vi "U-751 XY Stage Engine.vi"(0 "Notifier Name":string, 11 "COM Port":string[](array[string])) -> ()   [LabVIEW 2016]
uses:
  Stages Controls/Stage Notifier Element.ctl
  Stages Controls/Stage Actions.ctl
  Stages Controls/Stage Status.ctl
panel:
  in  "Quit":bool
  in  "Halt":bool
  in  "Home":bool
  in  "Get Position":bool
  in  "Y Position (µm)":dbl format="%#_4g"
  in  "X Position (µm)":dbl format="%#_4g"
  in  "XY Step Size (µm)":dbl format="%#_4g"
  in  "Up":bool
  in  "Down":bool
  in  "Left":bool
  in  "Right":bool
  in  "ReInitialize":bool
  in  "Error":bool
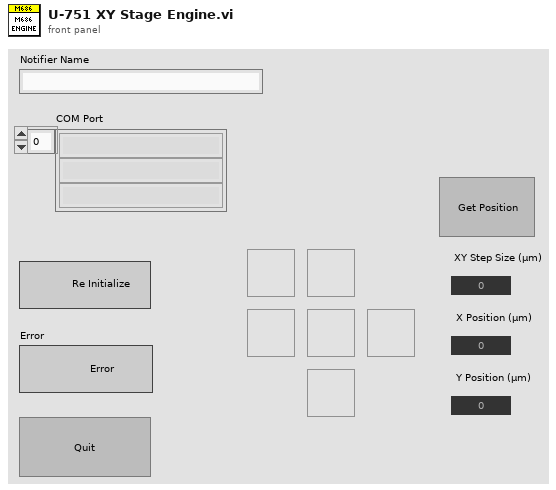
[diagram p1: front panel]
types:
  T1 = typedef "Stage Notifier Element.ctl" = cluster{"Action":T2, "Axis":bool[], "Setpoint":dbl[], "Velocity":dbl, "Cmd Recvd?":bool, "Position":dbl[], "Status":T3, "Misc":variant}
  T2 = typedef "Stage Actions.ctl" = enum16{"Get Position", "MVR", "MOVE", "HALT", "ONTARGET", "ERROR", "REFERENCE", "INIT", "VELOCITY", "STATUS", "EXIT", "HOME", "ZEROPOS", "NANOPOS", "ANALOG", "QUIT"}
  T3 = typedef "Stage Status.ctl" = enum16{"Error", "Abort", "Busy", "On Target"}
  T4 = enum32{"Invalid", "Standard", "Closed", "Hidden", "Minimized", "Maximized"}
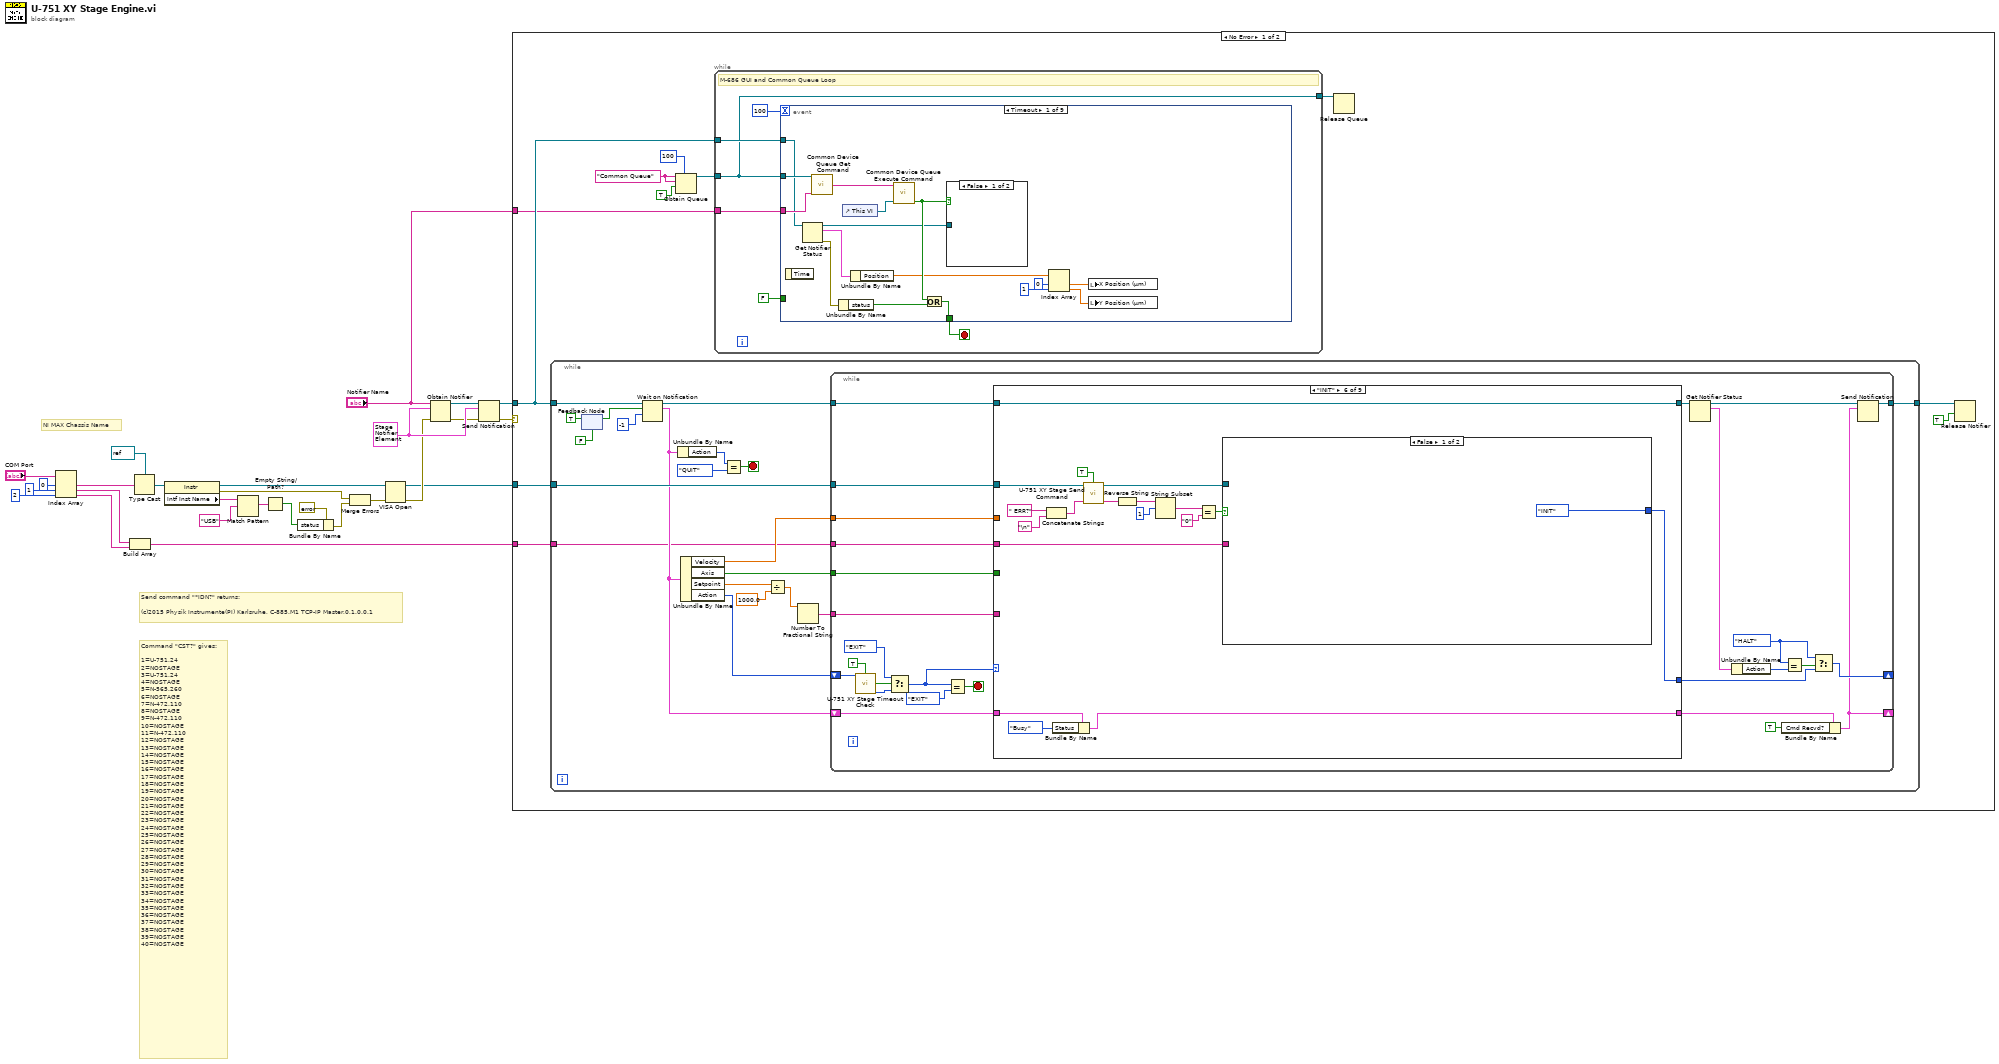
[diagram p0: block diagram]
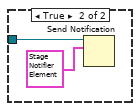
[diagram p2: hidden frame]
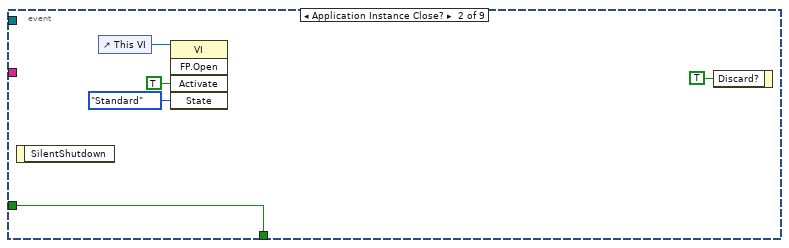
[diagram p3: hidden frame]
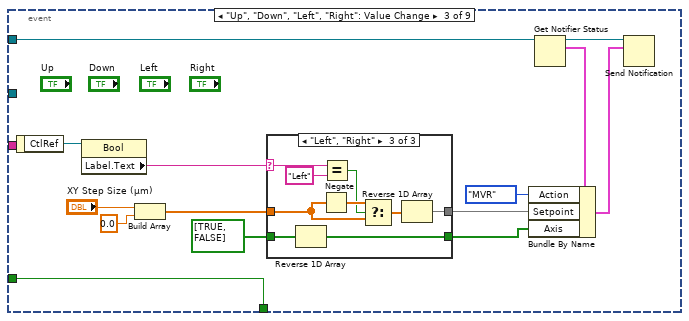
[diagram p4: hidden frame]
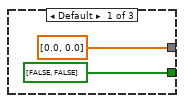
[diagram p5: hidden frame]
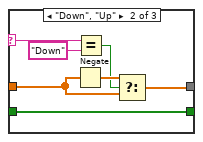
[diagram p6: hidden frame]
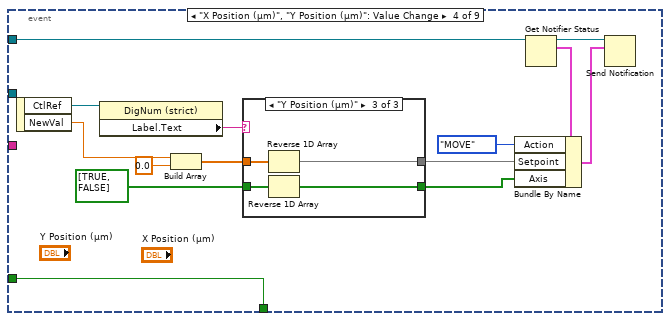
[diagram p7: hidden frame]
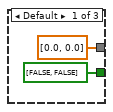
[diagram p8: hidden frame]
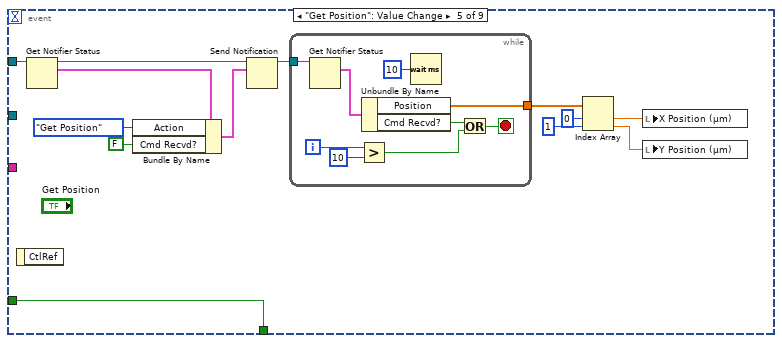
[diagram p10: hidden frame]
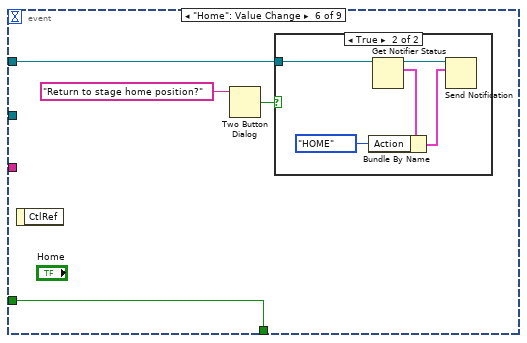
[diagram p11: hidden frame]
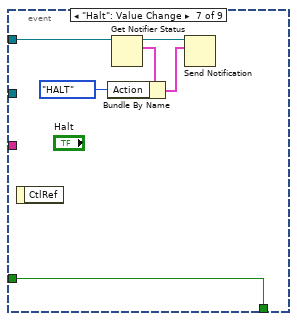
[diagram p13: hidden frame]
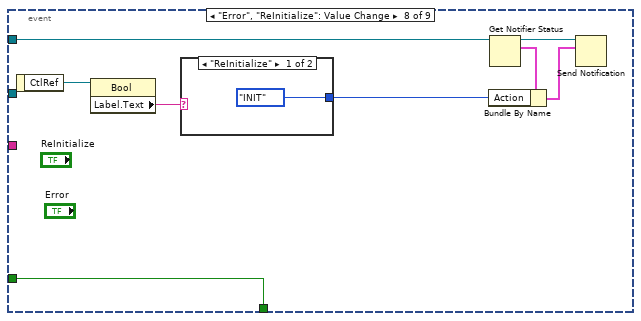
[diagram p14: hidden frame]
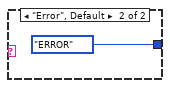
[diagram p15: hidden frame]
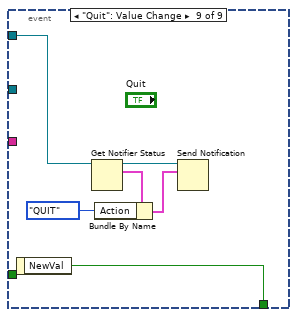
[diagram p16: hidden frame]
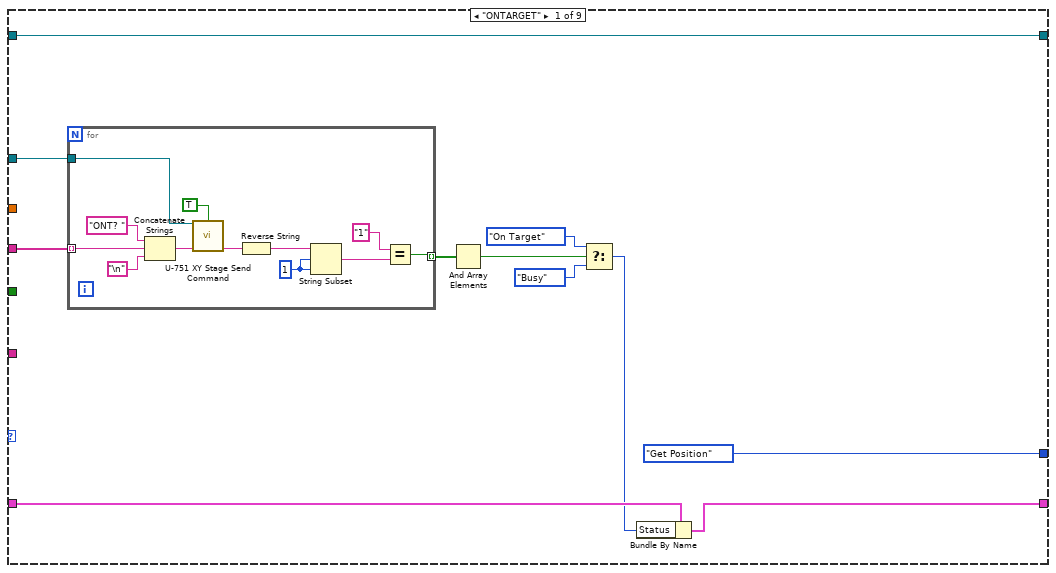
[diagram p17: hidden frame]
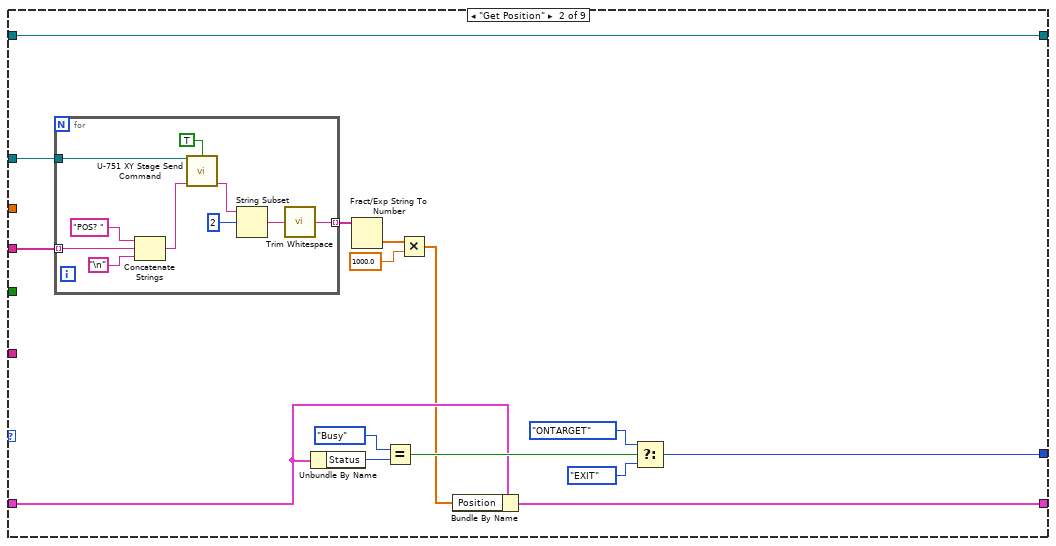
[diagram p18: hidden frame]
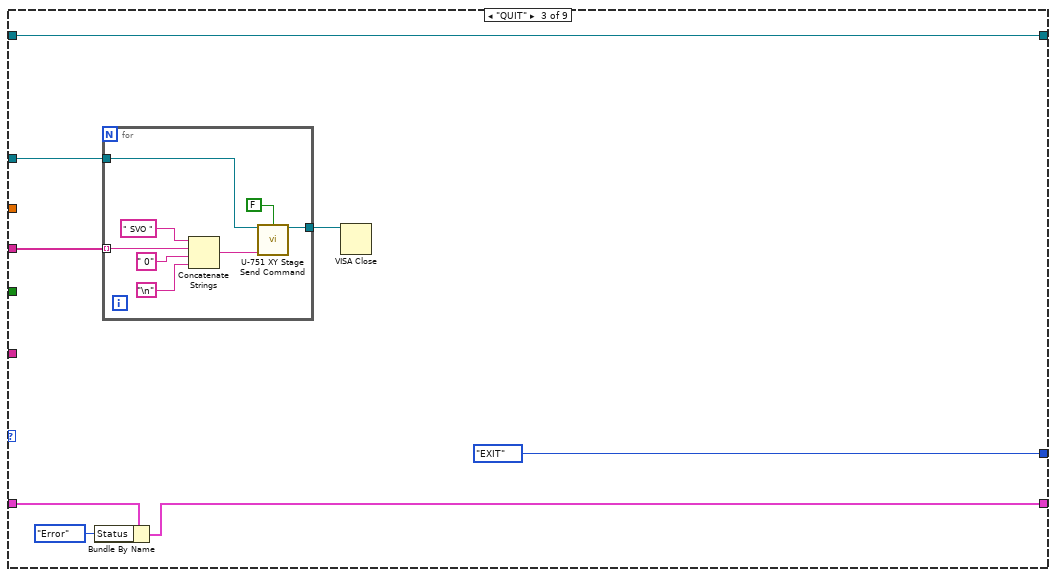
[diagram p19: hidden frame]
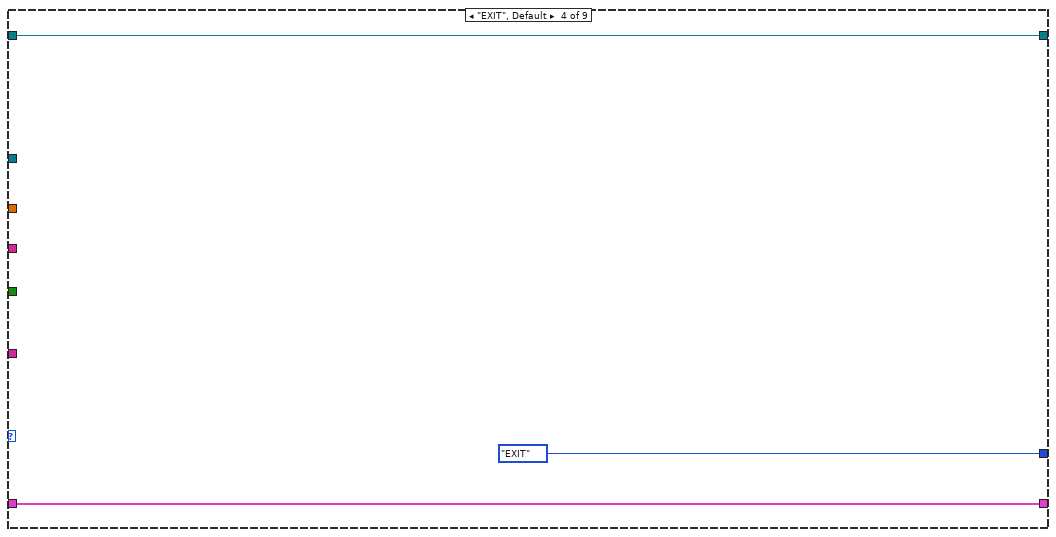
[diagram p20: hidden frame]
diagram:
  w14 = T1 {"Action"=enum."INIT", "Axis"=[], "Setpoint"=[], "Velocity"=0.5, "Cmd Recvd?"=FALSE, "Position"=[], "Status"=enum."Busy", "Misc"=variant} ("Stage Status")
  # "Command \"CST?\" gives:\n\n1=U-751.24 \n2=NOSTAGE \n3=U-751.24 \n4=NOSTAGE \n5=N-565.260 \n6=NOSTAGE \n7=N-472.110 \n8=NOSTAGE \n9=N-472.110 \n10=NOSTAGE \n11=N-472.110 \n12=NOSTAGE \n13=NOSTAGE \n14=NOSTAGE \n15=NOSTAGE \n16=NOSTAGE \n17=NOSTAGE \n18=NOSTAGE \n19=NOSTAGE \n20=NOSTAGE \n21=NOSTAGE \n22=NOSTAGE \n23=NOSTAGE \n24=NOSTAGE \n25=NOSTAGE \n26=NOSTAGE \n27=NOSTAGE \n28=NOSTAGE \n29=NOSTAGE \n30=NOSTAGE \n31=NOSTAGE \n32=NOSTAGE \n33=NOSTAGE \n34=NOSTAGE \n35=NOSTAGE \n36=NOSTAGE \n37=NOSTAGE \n38=NOSTAGE \n39=NOSTAGE \n40=NOSTAGE"
  # "Send command \"*IDN?\" returns:\n\n(c)2015 Physik Instrumente(PI) Karlsruhe, C-885.M1 TCP-IP Master,0,1.0.0.1"
  # "NI MAX Chassis Name"
  n1 = Index Array(array="COM Port", index #1=0 ("index"), index #2=1 ("index"), index #3=2 ("index")) -> (element #1=w20:string, element #2=w7:string, element #3=w6:string)
  n2 = Build Array(w7, w6) -> (w5:string[])
  n3 = Type Cast(type=refnum<visa-resource-name> refnum ("reference out"), x=w20) -> (*(type *) &x=w18:refnum<visa-resource-name>)
  n4 = property class="Instr"(reference=w18) -> (reference out=w4:refnum<visa-resource-name>, error out=w23:errorcluster, "Intf Inst Name"=w25:string)  [unwired: 1 in]
  n5 = Match Pattern(string=w25, regular expression="USB") -> (match substring=w27:string)  [unwired: 1 in, 3 out]
  n6 = Empty String/Path?(string/path=w27) -> (empty?=w24:bool)
  n7 = Bundle By Name(cluster=errorcluster {"status"=FALSE, "code"=0, "source"=""} ("Error"), "status"=w24) -> (w22:errorcluster)
  n8 = Merge Errors(w23, w22) -> (w3:errorcluster)
  n9 = VISA Open(error in (no error)=w3, VISA resource name=w4) -> (VISA resource name=w1:refnum<visa-resource-name>, error out=w2:errorcluster)  [unwired: 3 in]
  n10 = Obtain Notifier(name (unnamed)="Notifier Name", notification data type=w14, error in (no error)=w2) -> (notifier out=w15:refnum<notifier>, error out=w13:errorcluster)  [unwired: 1 in, 1 out]
  n11 = Send Notification(notification=w14, notifier=w15, error in (no error)=w13) -> (notifier out=w12:refnum<notifier>, error out=w11:errorcluster)
  n12 = case shown="No Error" w11 {
    selector: w11 -> [_ w453]
    tunnel: w1 -> [w38 w454]
    tunnel: w12 -> [w31 w455]
    tunnel: "Notifier Name" -> [w30 _]
    tunnel: w5 -> [w28 _]
    frame No Error {
      w34 = "Common Queue" ("Unique Notifier Name")
      n13 = while {
        tunnel: w31 -> [w192]
        tunnel: w38 -> [w182]
        tunnel: [w179] -> w37
        tunnel: w28 -> [w175]
        stop <- w194 stop-if-true
        n14 = feedback-in #1(TRUE) -> ()
        n15 = feedback #1(FALSE) -> (w176:bool)
        n16 = Wait on Notification(notifier=w192, ignore previous (F)=w176, timeout in ms (-1)=-1) -> (notifier out=w181:refnum<notifier>, notification=w180:T1)  [unwired: 1 in, 2 out]
        n17 = Unbundle By Name(w180) -> ("Action"=w191:T2)
        n18 = Unbundle By Name(w180) -> ("Velocity"=w188:dbl, "Axis"=w187:bool[], "Setpoint"=w184:dbl[], "Action"=w186:T2)
        n19 = Equal?(x=w191, y=Stage_Actions."QUIT") -> (x = y?=w194:bool)
        n20 = Divide(x=w184, y=1000.0) -> (x/y=w185:dbl[])
        n21 = Number To Fractional String(number=w185) -> (F-format string=w189:string[])  [unwired: 3 in]
        n22 = while {
          tunnel: w175 -> [w221]
          shift-right: [w214] -> _
          shift-left: w186 -> [w211]
          tunnel: w187 -> [w218]
          tunnel: w188 -> [w217]
          tunnel: w189 -> [w219]
          shift-right: [w197] -> _
          shift-left: w180 -> [w216]
          tunnel: w182 -> [w220]
          tunnel: w181 -> [w196]
          tunnel: [w200] -> w179
          stop <- w212 stop-if-true
          w203 = Stage_Actions."HALT" ("Action")
          n23 = call "U-751 XY Stage Timeout Check.vi"("Action"=w211, "User Input?"=TRUE) -> ("Timeout?"=w210:bool, "Action (Dup)"=w208:T2)  [unwired: 12 in]
          n24 = Select(t=Stage_Actions."EXIT" ("y"), s=w210, f=w208) -> (s? t:f=w207:T2)
          n25 = Equal?(x=w207, y=Stage_Actions."EXIT") -> (x = y?=w212:bool)
          n26 = case shown="\"INIT\"" w207 {
            selector: w207 -> [_ _ _ _ _ _ _ _ w411]
            tunnel: w221 -> [w230 w258 w276 _ _ w323 w362 w396 w423]
            tunnel: w220 -> [w232 w259 w277 _ w293 w314 w361 w391 w417]
            tunnel: w219 -> [_ _ _ _ _ _ _ _ w414]
            tunnel: w218 -> [_ _ _ _ _ _ _ _ w405]
            tunnel: w217 -> [_ _ _ _ _ _ _ _ w422]
            tunnel: [Stage_Actions."Get Position" ("Action") w256 Stage_Actions."EXIT" ("Action") Stage_Actions."EXIT" ("Action") w303 w322 w357 Stage_Actions."EXIT" ("Action") Stage_Actions."ONTARGET" ("Action")] -> w215
            tunnel: w216 -> [w225 w253 w274 w288 w301 w324 w355 w393 w419]
            tunnel: [w223 w251 w272 w288 w302 w325 w354 w392 w418] -> w199
            tunnel: w196 -> [w222 w245 w270 w286 w289 w309 w353 w390 w403]
            tunnel: [w222 w245 w270 w286 w289 w309 w353 w390 w403] -> w195
            frame "ONTARGET" {
              n27 = for {
                tunnel: [w242] -> w231 mode=indexing
                tunnel: w230 -> [w237] mode=indexing
                tunnel: w232 -> [w234]
                w238 = 1 ("length (rest)")
                n28 = Concatenate Strings("ONT? " ("string"), w237, "\n") -> (w236:string)
                n29 = call "U-751 XY Stage Send Command.vi"("VISA Ref"=w234, "Wait for Reply?"=TRUE, "Command"=w236) -> ("Response"=w233:string)  [unwired: 10 in, 2 out]
                n30 = Reverse String(1:w233) -> (0:w239:string)
                n31 = String Subset(string=w239, offset (0)=w238, length (rest)=w238) -> (substring=w244:string)
                n32 = Equal?(x="1", y=w244) -> (x = y?=w242:bool)
              }
              n33 = And Array Elements(Boolean array=w231) -> (logical AND=w226:bool)
              n34 = Select(t=Stage_Status."On Target" ("Status"), s=w226, f=Stage_Status."Busy" ("Status")) -> (s? t:f=w224:T3)
              n35 = Bundle By Name(cluster=w225, "Status"=w224) -> (w223:T1)
            }
            frame "Get Position" {
              n36 = for {
                tunnel: [w269] -> w257 mode=indexing
                tunnel: w258 -> [w264] mode=indexing
                tunnel: w259 -> [w263]
                n37 = Concatenate Strings("POS? " ("string"), w264, "\n") -> (w262:string)
                n38 = call "U-751 XY Stage Send Command.vi"("VISA Ref"=w263, "Wait for Reply?"=TRUE, "Command"=w262) -> ("Response"=w260:string)  [unwired: 10 in, 2 out]
                n39 = String Subset(string=w260, offset (0)=2) -> (substring=w265:string)  [unwired: 1 in]
                n40 = call <vilib>:"Trim Whitespace.vi"("string"=w265) -> ("trimmed string"=w269:string)  [unwired: 1 in]
              }
              n41 = Unbundle By Name(w253) -> ("Status"=w252:T3)
              n42 = Fract/Exp String To Number(string=w257) -> (number=w250:dbl[])  [unwired: 3 in, 1 out]
              n43 = Equal?(x=Stage_Status."Busy", y=w252) -> (x = y?=w254:bool)
              n44 = Multiply(x=w250, y=1000.0) -> (x*y=w247:dbl[])
              n45 = Bundle By Name(cluster=w253, "Position"=w247) -> (w251:T1)
              n46 = Select(t=Stage_Actions."ONTARGET" ("Action"), s=w254, f=Stage_Actions."EXIT" ("Action")) -> (s? t:f=w256:T2)
            }
            frame "QUIT" {
              n47 = Bundle By Name(cluster=w274, "Status"=Stage_Status."Error") -> (w272:T1)
              n48 = for {
                tunnel: w277 -> [w279]
                tunnel: w276 -> [w282] mode=indexing
                tunnel: [w278] -> w271
                n49 = Concatenate Strings(" SVO " ("string"), w282, " 0" ("string"), "\n") -> (w281:string)
                n50 = call "U-751 XY Stage Send Command.vi"("VISA Ref"=w279, "Wait for Reply?"=FALSE, "Command"=w281) -> ("VISA Ref Out"=w278:refnum<visa-resource-name>)  [unwired: 10 in, 2 out]
              }
              n51 = VISA Close(VISA resource name=w271) -> ()  [unwired: 1 in, 1 out]
            }
            frame "EXIT", Default {
            }
            frame "ERROR" {
              n52 = Concatenate Strings(" ERR?" ("string"), "\n") -> (w291:string)
              n53 = call "U-751 XY Stage Send Command.vi"("VISA Ref"=w293, "Wait for Reply?"=TRUE, "Command"=w291) -> ("Response"=w290:string)  [unwired: 10 in, 2 out]
              n54 = Reverse String(1:w290) -> (0:w298:string)
              n55 = String Subset(string=w298, offset (0)=1) -> (substring=w300:string)  [unwired: 1 in]
              n56 = Equal?(x=w300, y="0") -> (x = y?=w294:bool)
              n57 = Select(t=Stage_Status."Busy" ("Status"), s=w294, f=Stage_Status."Error" ("Status")) -> (s? t:f=w306:T3)
              n58 = Bundle By Name(cluster=w301, "Status"=w306) -> (w302:T1)
              n59 = Select(t=Stage_Actions."ONTARGET" ("Action"), s=w294, f=Stage_Actions."ERROR") -> (s? t:f=w303:T2)
            }
            frame "INIT" {
              n60 = Concatenate Strings(" ERR?" ("string"), "\n") -> (w311:string)
              n61 = Bundle By Name(cluster=w324, "Status"=Stage_Status."Busy") -> (w325:T1)
              n62 = call "U-751 XY Stage Send Command.vi"("VISA Ref"=w314, "Wait for Reply?"=TRUE, "Command"=w311) -> ("VISA Ref Out"=w313:refnum<visa-resource-name>, "Response"=w310:string)  [unwired: 10 in, 1 out]
              n63 = Reverse String(1:w310) -> (0:w320:string)
              n64 = String Subset(string=w320, offset (0)=1) -> (substring=w318:string)  [unwired: 1 in]
              n65 = Equal?(x=w318, y="0") -> (x = y?=w315:bool)
              n66 = case shown="False" w315 {
                tunnel: w323 -> [_ w334]
                tunnel: [Stage_Actions."INIT" ("Action") w332] -> w322
                tunnel: w313 -> [_ w329]
                frame False {
                }
                frame True {
                  n67 = for {
                    tunnel: w334 -> [w348] mode=indexing
                    tunnel: w329 -> [w341]
                    tunnel: [w343] -> w328 mode=indexing
                    w347 = 1 ("length (rest)")
                    n68 = Concatenate Strings(" SVO " ("string"), w348, " 1" ("string"), "\n") -> (w340:string)
                    n69 = Concatenate Strings(" SVO? " ("string"), w348, "\n") -> (w337:string)
                    n70 = call "U-751 XY Stage Send Command.vi"("VISA Ref"=w341, "Wait for Reply?"=FALSE, "Command"=w340) -> ("VISA Ref Out"=w338:refnum<visa-resource-name>)  [unwired: 10 in, 2 out]
                    n71 = call "U-751 XY Stage Send Command.vi"("VISA Ref"=w338, "Wait for Reply?"=TRUE, "Command"=w337) -> ("Response"=w335:string)  [unwired: 10 in, 2 out]
                    n72 = Reverse String(1:w335) -> (0:w346:string)
                    n73 = String Subset(string=w346, offset (0)=w347, length (rest)=w347) -> (substring=w345:string)
                    n74 = Equal?(x=w345, y="1") -> (x = y?=w343:bool)
                  }
                  n75 = And Array Elements(Boolean array=w328) -> (logical AND=w330:bool)
                  n76 = Select(t=Stage_Actions."REFERENCE" ("Action"), s=w330, f=Stage_Actions."INIT" ("Action")) -> (s? t:f=w332:T2)
                }
              }
            }
            frame "REFERENCE" {
              n77 = for {
                tunnel: w362 -> [w387] mode=indexing
                tunnel: w361 -> [w381]
                tunnel: [w380] -> w358
                tunnel: [w382] -> w360 mode=indexing
                w385 = 1 ("length (rest)")
                n78 = Concatenate Strings(" FRF? " ("string"), w387, "\n") -> (w379:string)
                n79 = call "U-751 XY Stage Send Command.vi"("VISA Ref"=w381, "Wait for Reply?"=TRUE, "Command"=w379) -> ("VISA Ref Out"=w380:refnum<visa-resource-name>, "Response"=w378:string)  [unwired: 10 in, 1 out]
                n80 = Reverse String(1:w378) -> (0:w386:string)
                n81 = String Subset(string=w386, offset (0)=w385, length (rest)=w385) -> (substring=w383:string)
                n82 = Equal?(x=w383, y="1") -> (x = y?=w382:bool)
              }
              n83 = Bundle By Name(cluster=w355, "Status"=Stage_Status."Busy") -> (w354:T1)
              n84 = And Array Elements(Boolean array=w360) -> (logical AND=w359:bool)
              n85 = case shown="False" w359 {
                tunnel: w358 -> [w364 _]
                tunnel: [w363 Stage_Actions."ONTARGET" ("Action")] -> w357
                frame False {
                  n86 = Two Button Dialog(message="M686", 1:"Skip" ("F button name (\"Cancel\")"), 2:"Reference" ("T button name (\"OK\")")) -> (T button?=w368:bool)
                  n87 = case shown="True" w368 {
                    tunnel: [Stage_Actions."HALT" ("Action") Stage_Actions."ONTARGET" ("Action")] -> w363
                    tunnel: w364 -> [_ w372]
                    frame False {
                    }
                    frame True {
                      n88 = Concatenate Strings("FRF" ("string"), "\n") -> (w371:string)
                      n89 = call "U-751 XY Stage Send Command.vi"("VISA Ref"=w372, "Wait for Reply?"=FALSE, "Command"=w371) -> ()  [unwired: 10 in, 3 out]
                    }
                  }
                }
                frame True {
                }
              }
            }
            frame "HALT" {
              n90 = for {
                tunnel: w396 -> [w400] mode=indexing
                tunnel: w391 -> [w398]
                n91 = Concatenate Strings(w400, " HLT" ("string"), "\n") -> (w399:string)
                n92 = call "U-751 XY Stage Send Command.vi"("VISA Ref"=w398, "Wait for Reply?"=FALSE, "Command"=w399) -> ()  [unwired: 10 in, 3 out]
              }
              n93 = Bundle By Name(cluster=w393, "Status"=Stage_Status."Abort") -> (w392:T1)
            }
            frame "MVR", "MOVE", "HOME" {
              n94 = Bundle By Name(cluster=w419, "Status"=Stage_Status."Busy") -> (w418:T1)
              n95 = Equal?(x=Stage_Actions."MVR", y=w411) -> (x = y?=w404:bool)
              n96 = Equal?(x=w411, y=Stage_Actions."HOME") -> (x = y?=w415:bool)
              n97 = Not(x=w415) -> (.not. x?=w410:bool)
              n98 = Select(t="MVR ", s=w404, f="MOV ") -> (s? t:f=w406:string)
              n99 = Select(t=w414, s=w410, f=string[] ["12.5", "12.5"]) -> (s? t:f=w413:string[])
              n100 = for {
                tunnel: w423 -> [w429] mode=indexing
                tunnel: w413 -> [w428] mode=indexing
                tunnel: w405 -> [w427] mode=indexing
                tunnel: w422 -> [w426]
                tunnel: w417 -> [w425]
                tunnel: w406 -> [w424]
                n101 = case shown="True" w427 {
                  tunnel: w429 -> [_ w437]
                  tunnel: w428 -> [_ w438]
                  tunnel: w425 -> [_ w431]
                  tunnel: w426 -> [_ w436]
                  tunnel: w424 -> [_ w430]
                  frame False {
                  }
                  frame True {
                    n102 = Equal To 0?(x=w436) -> (x = 0?=w435:bool)
                    n103 = call <vilib>:"Space Constant.vi"() -> ("String"=w439:string)
                    n104 = case shown="False" w435 {
                      tunnel: w437 -> [w447 _]
                      tunnel: w436 -> [w444 _]
                      tunnel: [w446 ""] -> w434
                      frame False {
                        n105 = Number To Fractional String(number=w444) -> (F-format string=w445:string)  [unwired: 3 in]
                        n106 = call <vilib>:"Space Constant.vi"() -> ("String"=w450:string)
                        n107 = Concatenate Strings("VEL ", w447, w450, w445, "\n") -> (w446:string)
                      }
                      frame True {
                      }
                    }
                    n108 = Concatenate Strings(w430, w437, w439, w438, "\n") -> (w433:string)
                    n109 = Build Array(w434, w433) -> (w432:string[])
                    n110 = for {
                      tunnel: w432 -> [w443] mode=indexing
                      tunnel: w431 -> [w441]
                      n111 = call "U-751 XY Stage Send Command.vi"("VISA Ref"=w441, "Wait for Reply?"=FALSE, "Command"=w443) -> ()  [unwired: 10 in, 3 out]
                    }
                  }
                }
              }
            }
          }
          n112 = Get Notifier Status(notifier=w195) -> (notifier out=w201:refnum<notifier>, current notification=w202:T1)  [unwired: 1 in, 3 out]
          n113 = Unbundle By Name(w202) -> ("Action"=w204:T2)
          n114 = Bundle By Name(cluster=w199, "Cmd Recvd?"=TRUE) -> (w197:T1)
          n115 = Equal?(x=w203, y=w204) -> (x = y?=w205:bool)
          n116 = Select(t=w203, s=w205, f=w215) -> (s? t:f=w214:T2)
          n117 = Send Notification(notification=w197, notifier=w201) -> (notifier out=w200:refnum<notifier>)  [unwired: 1 in, 1 out]
        }
      }
      n118 = Obtain Queue(max queue size (-1, unlimited)=100, name (unnamed)=w34, element data type=w34, create if not found? (T)=TRUE) -> (queue out=w35:refnum<queue>)  [unwired: 1 in, 2 out]
      n119 = while {
        tunnel: w35 -> [w39]
        tunnel: w30 -> [w42]
        tunnel: w31 -> [w43]
        tunnel: [w39] -> w29
        stop <- w41 stop-if-true
        # "M-686 GUI and Common Queue Loop"
        n120 = event shown="[0] Timeout" {
          selector: _ -> [_ _ _ _ _ _ _ _ _]
          dyn-events: _ -> [_ _ _ _ _ _ _ _ _]
          timeout: 100 -> [_ _ _ _ _ _ _ _ _]
          tunnel: w39 -> [w54 _ _ _ _ _ _ _ _]
          tunnel: w43 -> [w51 _ w74 w106 w133 w144 w157 w163 w174]
          tunnel: w42 -> [w53 _ _ _ _ _ _ _ _]
          tunnel: [w52 w67 w77 w113 w134 w146 w158 w166 w170] -> w41
          tunnel: FALSE -> [_ w67 w77 w113 w134 w146 w158 w166 _]
          event Timeout {
            n121 = event-data() -> ()  [unwired: 1 in, 1 out]
            n122 = Get Notifier Status(notifier=w51) -> (notifier out=w55:refnum<notifier>, current notification=w50:T1, error out=w60:errorcluster)  [unwired: 1 in, 2 out]
            n123 = call "Common Device Queue Get Command.vi"("Common Queue"=w54, "Notifier Name"=w53) -> ("Command"=w59:string)  [unwired: 12 in, 1 out]
            n124 = Unbundle By Name(w60) -> ("status"=w57:bool)
            n125 = control-ref of="This VI"() -> (w58:refnum<vi>)
            n126 = Unbundle By Name(w50) -> ("Position"=w45:dbl[])
            n127 = call "Common Device Queue Execute Command.vi"("Common Command"=w59, "VI Refnum"=w58) -> ("Quit?"=w56:bool)  [unwired: 12 in, 1 out]
            n128 = Or(x=w56, y=w57) -> (x .or. y?=w52:bool)
            n129 = case shown="False" w56 {
              tunnel: w55 -> [_ w62]
              frame False {
              }
              frame True {
                n130 = Send Notification(notification=T1 {"Action"=enum."QUIT", "Axis"=[], "Setpoint"=[], "Velocity"=0.5, "Cmd Recvd?"=FALSE, "Position"=[], "Status"=enum."Error", "Misc"=variant} ("Stage Status"), notifier=w62) -> ()  [unwired: 1 in, 2 out]
              }
            }
            n131 = Index Array(array=w45, index #1=0 ("index"), index #2=1 ("index")) -> (element #1=w49:dbl, element #2=w48:dbl)
            n132 = local write "X Position (µm)"(w49) -> ()
            n133 = local write "Y Position (µm)"(w48) -> ()
          }
          event Application Instance Close? {
            n134 = event-data() -> ()  [unwired: 1 in, 1 out]
            n135 = control-ref of="This VI"() -> (w64:refnum<vi>)
            n136 = invoke class="VI" method="FP.Open"(reference=w64, "Activate"=TRUE ("Activate?"), "State"=T4."Standard") -> ()  [unwired: 2 in, 5 out]
            n137 = event-data("Discard?"=TRUE) -> ()  [unwired: 1 in, 1 out]
          }
          event "Up", "Down", "Left", "Right": Value Change {
            n138 = event-data() -> ("CtlRef"=w76:refnum<vi>)  [unwired: 1 in]
            n139 = property class="Bool"(reference=w76) -> ("Label.Text"=w81:string)  [unwired: 1 in, 2 out]
            n140 = Build Array("XY Step Size (µm)", 0.0 ("element")) -> (w79:dbl[])
            n141 = case shown="\"Left\", \"Right\"" w81 {
              selector: w81 -> [_ w90 w96]
              tunnel: w79 -> [_ w87 w95]
              tunnel: bool[] [TRUE, FALSE] -> [_ w84 w93]
              tunnel: [dbl[] [0.0, 0.0] w86 w92] -> w72
              tunnel: [bool[] [FALSE, FALSE] w84 w91] -> w71
              frame Default {
              }
              frame "Down", "Up" {
                n142 = Negate(x=w87) -> (-x=w88:dbl[])
                n143 = Equal?(x=w90, y="Down") -> (x = y?=w85:bool)
                n144 = Select(t=w88, s=w85, f=w87) -> (s? t:f=w86:dbl[])
              }
              frame "Left", "Right" {
                n145 = Reverse 1D Array(array=w93) -> (reversed array=w91:bool[])
                n146 = Negate(x=w95) -> (-x=w98:dbl[])
                n147 = Equal?(x=w96, y="Left") -> (x = y?=w97:bool)
                n148 = Select(t=w98, s=w97, f=w95) -> (s? t:f=w94:dbl[])
                n149 = Reverse 1D Array(array=w94) -> (reversed array=w92:dbl[])
              }
            }
            n150 = Get Notifier Status(notifier=w74) -> (notifier out=w69:refnum<notifier>, current notification=w73:T1)  [unwired: 1 in, 3 out]
            n151 = Bundle By Name(cluster=w73, "Action"=Stage_Actions."MVR", "Setpoint"=w72, "Axis"=w71) -> (w68:T1)
            n152 = Send Notification(notification=w68, notifier=w69) -> ()  [unwired: 1 in, 2 out]
          }
          event "X Position (µm)", "Y Position (µm)": Value Change {
            n153 = event-data() -> ("CtlRef"=w108:refnum<vi>, "NewVal"=w107:dbl)  [unwired: 1 in]
            n154 = property class="DigNum (strict)"(reference=w108) -> ("Label.Text"=w111:string)  [unwired: 1 in, 2 out]
            n155 = Build Array(w107, 0.0 ("element")) -> (w112:dbl[])
            n156 = case shown="\"Y Position (µm)\"" w111 {
              tunnel: w112 -> [_ w117 w121]
              tunnel: bool[] [TRUE, FALSE] -> [_ w116 w120]
              tunnel: [dbl[] [0.0, 0.0] w117 w119] -> w103
              tunnel: [bool[] [FALSE, FALSE] w116 w118] -> w102
              frame Default {
              }
              frame "X Position (µm)" {
              }
              frame "Y Position (µm)" {
                n157 = Reverse 1D Array(array=w121) -> (reversed array=w119:dbl[])
                n158 = Reverse 1D Array(array=w120) -> (reversed array=w118:bool[])
              }
            }
            n159 = Get Notifier Status(notifier=w106) -> (notifier out=w105:refnum<notifier>, current notification=w104:T1)  [unwired: 1 in, 3 out]
            n160 = Bundle By Name(cluster=w104, "Action"=Stage_Actions."MOVE", "Setpoint"=w103, "Axis"=w102) -> (w100:T1)
            n161 = Send Notification(notification=w100, notifier=w105) -> ()  [unwired: 1 in, 2 out]
          }
          event "Get Position": Value Change {
            n162 = event-data() -> ()  [unwired: 1 in, 1 out]
            n163 = Get Notifier Status(notifier=w133) -> (notifier out=w132:refnum<notifier>, current notification=w131:T1)  [unwired: 1 in, 3 out]
            n164 = Bundle By Name(cluster=w131, "Action"=Stage_Actions."Get Position", "Cmd Recvd?"=FALSE) -> (w128:T1)
            n165 = Send Notification(notification=w128, notifier=w132) -> (notifier out=w127:refnum<notifier>)  [unwired: 1 in, 1 out]
            n166 = while {
              tunnel: w127 -> [w143]
              tunnel: [w135] -> w126
              i -> [w139]
              stop <- w136 stop-if-true
              n167 = Get Notifier Status(notifier=w143) -> (current notification=w142:T1)  [unwired: 1 in, 4 out]
              n168 = Greater?(x=w139, y=10) -> (0:w137:bool)
              n169 = Unbundle By Name(w142) -> ("Position"=w135:dbl[], "Cmd Recvd?"=w138:bool)
              n170 = Wait (ms)(milliseconds to wait=u32 10) -> ()  [unwired: 1 out]
              n171 = Or(x=w138, y=w137) -> (x .or. y?=w136:bool)
            }
            n172 = Index Array(array=w126, index #1=0 ("index"), index #2=1 ("index")) -> (element #1=w123:dbl, element #2=w122:dbl)
            n173 = local write "X Position (µm)"(w123) -> ()
            n174 = local write "Y Position (µm)"(w122) -> ()
          }
          event "Home": Value Change {
            n175 = event-data() -> ()  [unwired: 1 in, 1 out]
            n176 = Two Button Dialog(message="Return to stage home position?") -> (T button?=w145:bool)  [unwired: 2 in]
            n177 = case shown="True" w145 {
              tunnel: w144 -> [_ w152]
              frame False {
              }
              frame True {
                n178 = Get Notifier Status(notifier=w152) -> (notifier out=w151:refnum<notifier>, current notification=w150:T1)  [unwired: 1 in, 3 out]
                n179 = Bundle By Name(cluster=w150, "Action"=Stage_Actions."HOME") -> (w149:T1)
                n180 = Send Notification(notification=w149, notifier=w151) -> ()  [unwired: 1 in, 2 out]
              }
            }
          }
          event "Halt": Value Change {
            n181 = event-data() -> ()  [unwired: 1 in, 1 out]
            n182 = Get Notifier Status(notifier=w157) -> (notifier out=w156:refnum<notifier>, current notification=w155:T1)  [unwired: 1 in, 3 out]
            n183 = Bundle By Name(cluster=w155, "Action"=Stage_Actions."HALT") -> (w154:T1)
            n184 = Send Notification(notification=w154, notifier=w156) -> ()  [unwired: 1 in, 2 out]
          }
          event "Error", "ReInitialize": Value Change {
            n185 = event-data() -> ("CtlRef"=w165:refnum<vi>)  [unwired: 1 in]
            n186 = property class="Bool"(reference=w165) -> ("Label.Text"=w164:string)  [unwired: 1 in, 2 out]
            n187 = case shown="\"ReInitialize\"" w164 {
              tunnel: [Stage_Actions."INIT" ("Action") Stage_Actions."ERROR" ("Action")] -> w159
              frame "ReInitialize" {
              }
              frame "Error", Default {
              }
            }
            n188 = Get Notifier Status(notifier=w163) -> (notifier out=w162:refnum<notifier>, current notification=w161:T1)  [unwired: 1 in, 3 out]
            n189 = Bundle By Name(cluster=w161, "Action"=w159) -> (w160:T1)
            n190 = Send Notification(notification=w160, notifier=w162) -> ()  [unwired: 1 in, 2 out]
          }
          event "Quit": Value Change {
            n191 = event-data() -> ("NewVal"=w170:bool)  [unwired: 1 in]
            n192 = Get Notifier Status(notifier=w174) -> (notifier out=w173:refnum<notifier>, current notification=w172:T1)  [unwired: 1 in, 3 out]
            n193 = Bundle By Name(cluster=w172, "Action"=Stage_Actions."QUIT") -> (w171:T1)
            n194 = Send Notification(notification=w171, notifier=w173) -> ()  [unwired: 1 in, 2 out]
          }
        }
      }
      n195 = Release Queue(queue=w29) -> ()  [unwired: 2 in, 3 out]
      n196 = Release Notifier(notifier=w37, force destroy? (F)=TRUE) -> ()  [unwired: 1 in, 3 out]
    }
    frame Error {
      n197 = VISA Close(VISA resource name=w454, error in (no error)=w453) -> (error out=w452:errorcluster)
      n198 = Release Notifier(notifier=w455, force destroy? (F)=TRUE, error in (no error)=w452) -> (error out=w460:errorcluster)  [unwired: 2 out]
      n199 = Unbundle By Name(w460) -> ("source"=w457:string)
      n200 = Concatenate Strings("M-686 (XY Sample Stage) Initialization Error", "\r", w457) -> (w456:string)
      n201 = One Button Dialog(message=w456) -> ()  [unwired: 1 in, 1 out]
    }
  }
